vi "DiscArchiver.ProcDestructor.vi"(0 "i ref in":refnum<vi>, 5 "error in (no error)":errorcluster) -> (14 "i ref out":refnum<vi>, 19 "error out":errorcluster)   [LabVIEW 2014, in "DiscArchiver.lvlib"]
doc: "This is the counterpart to ProcConstructor and is called before the \"deactivate\" is called. This can be used to shutdown/deinitialize things."
uses:
  DiscArchiver.lvlib
  CSlibraries-extern/DimLVEvent/LVDimInterface/LVDimInterface.lvlib
  CSlibraries/UtilityLib/UtilityLib.lvlib
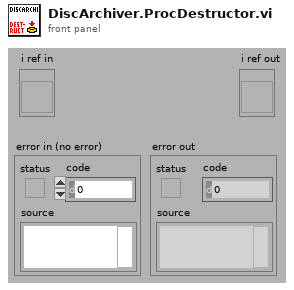
[diagram p1: front panel]
types:
  T1 = typedef "DiscArchiver.lvlib/DiscArchiver.i attribute.ctl" = cluster{"file prefix":string, "actual file":string, "nOfEvents":i32, "file":refnum<file>, "eventBuilder":string, "disc size alarm":bool, "dataDescription":string, "dataDescriptionURL":string, "eventDataURL":string, "headerID":dbl, "completeData":bool, "nOfEventsID":i32, "dataFileID":i32}
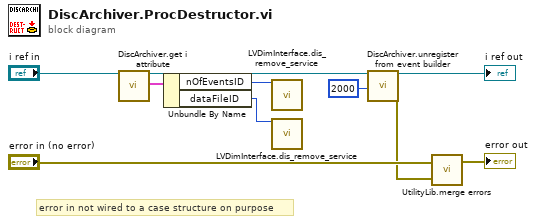
[diagram p0: block diagram]
diagram:
  # "error in not wired to a case structure on purpose"
  n1 = call "DiscArchiver.get i attribute.vi"("i ref in"="i ref in") -> ("i ref out"=w4:refnum<vi>, "i attribute"=w3:T1)  [unwired: 16 in, 1 out]
  n2 = Unbundle By Name(w3) -> ("nOfEventsID"=w2:i32, "dataFileID"=w1:i32)
  n3 = call "LVDimInterface.dis_remove_service.vi"("my_serviceID"=w2) -> ()  [unwired: 18 in, 1 out]
  n4 = call "LVDimInterface.dis_remove_service.vi"("my_serviceID"=w1) -> ()  [unwired: 18 in, 1 out]
  n5 = call "DiscArchiver.unregister from event builder.vi"("i ref in"=w4, "ms timeout (10000)"=2000 ("ms timeout (100)")) -> ("i ref out"=→"i ref out":refnum<vi>, "error out"=w5:errorcluster)  [unwired: 15 in, 1 out]
  n6 = call "UtilityLib.merge errors.vi"("error2 (no error)"=w5, "error1 (no error)"="error in (no error)") -> ("error out"=→"error out":errorcluster)
